vi "CVT2SaveAndReadTest.vi"() -> (3 "Unit Test Framework Results":T1)   [LabVIEW 2013, in "UnitTests.lvlib"]
uses:
  UnitTests.lvlib
  <vilib>/utf/common/utf_test_result_troll.ctl
  <vilib>/utf/common/utf_test_result.ctl
  <vilib>/utf/common/utf_test_result_failure.ctl
  <vilib>/utf/common/utf_test_comparison_operators.ctl
  <vilib>/utf/common/utf_vi_tag.ctl
  <vilib>/NI/Current Value Table/DataTypes/I32_Read Index.vi
  <vilib>/NI/Current Value Table/DataTypes/I32_Write Index.vi
  <vilib>/NI/Current Value Table/Memory Block.vi
  <vilib>/NI/Current Value Table/DataTypes/I32_Memory Block.vi
  <vilib>/utf/NI_UnitTestFramework.lvlib
  <vilib>/NI/Current Value Table/Current Value Table.lvlib
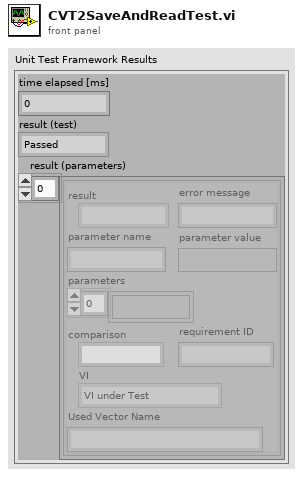
[diagram p1: front panel]
types:
  T1 = typedef "NI_UnitTestFramework.lvlib/utf_test_result_troll.ctl" = cluster{"time elapsed [ms]":u32, "result (test)":T2, "result (parameters)":T3[]}
  T2 = typedef "NI_UnitTestFramework.lvlib/utf_test_result.ctl" = enum16{"Passed", "Failed", "Error", "Skipped", "Not Processed"}
  T3 = typedef "NI_UnitTestFramework.lvlib/utf_test_result_failure.ctl" = cluster{"result":T2, "error message":string, "parameter name":string, "parameter value":variant, "parameters":variant[], "comparison":T4, "requirement ID":string, "VI":T5, "Used Vector Name":string}
  T4 = typedef "NI_UnitTestFramework.lvlib/utf_test_comparison_operators.ctl" = enum16{"=", "!=", ">", ">=", "<", "<=", "range", "symmetric tolerance", "asymmetric tolerance", "string contains", "string not contain", "array size", "string length", "array range", "by element", "array range (limit array)", "user-defined", "array contains", "array not contain", "vector length", "= (elm)", "!= (elm)", "= (case insensitive)", "!= (case insensitive)"}
  T5 = typedef "NI_UnitTestFramework.lvlib/utf_vi_tag.ctl" = enum16{"Setup VI", "VI under Test", "Teardown VI"}
  T6 = typedef "Current Value Table.lvlib/File Format.ctl" = cluster{"Tags":T7[], "Group Listings":T9[]}
  T7 = typedef "Current Value Table.lvlib/Single Tag.ctl" = cluster{"Data Type":T8, "Name":string, "Value":string, "Description":string}
  T8 = typedef "Current Value Table.lvlib/Data Types.ctl" = enum16{"Double", "Single", "I64", "I32", "I16", "I8", "U64", "U32", "U16", "U8", "String", "Boolean", "Array of U8", "Array of U16", "Array of U32", "Array of U64", "Array of I64", "Array of I32", "Array of I16", "Array of I8", "Array of Double", "Array of Single", "Array of Boolean", "Array of String"}
  T9 = typedef "Current Value Table.lvlib/Tag Grouping set.ctl" = cluster{"Group":string, "Tag Names":string[]}
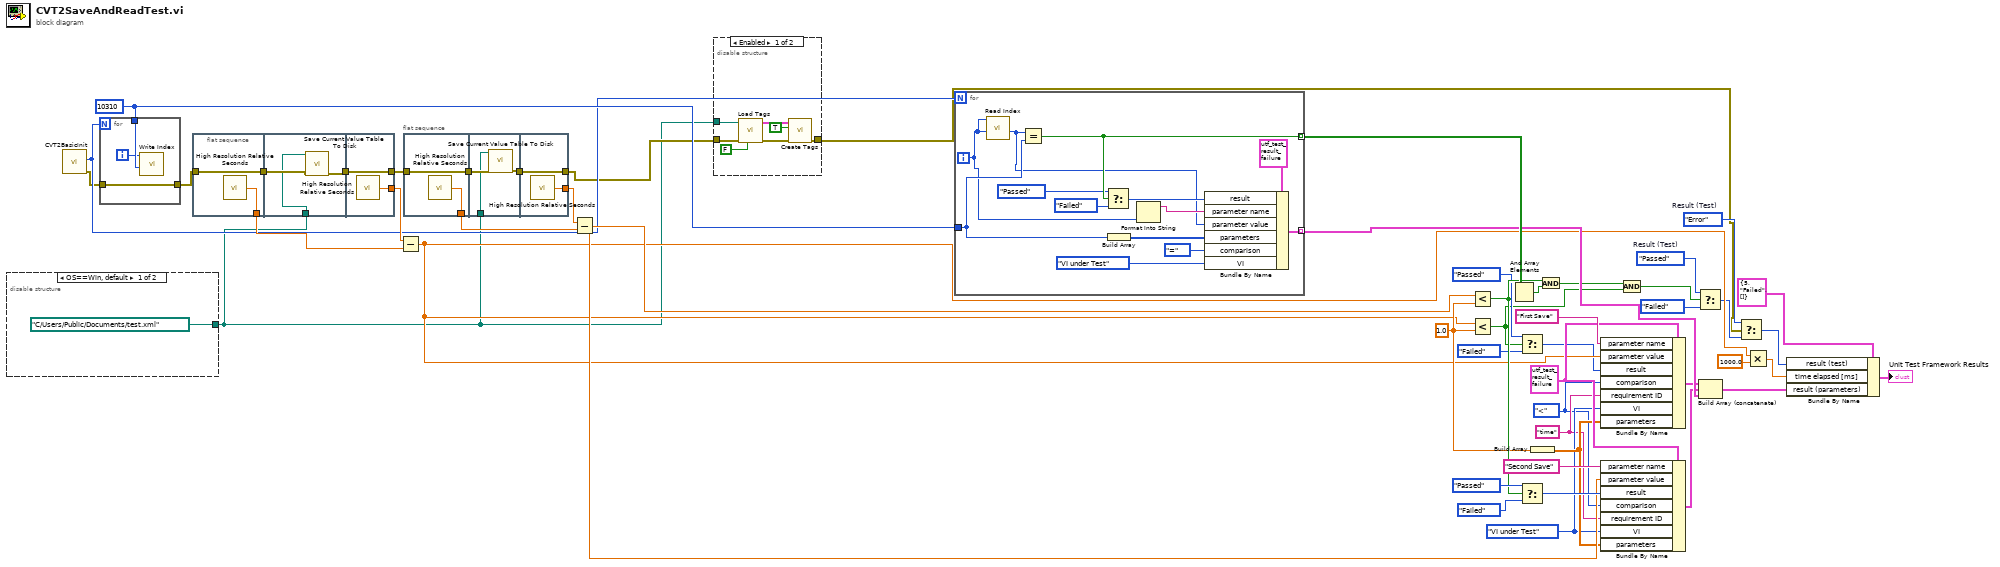
[diagram p0: block diagram]
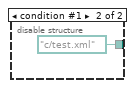
[diagram p3: hidden frame]
diagram:
  w29 = 10310 ("Value")
  w21 = T3 {"result"=enum."Passed", "error message"="", "parameter name"="", "parameter value"=variant, "parameters"=[], "comparison"=enum."=", "requirement ID"="", "VI"=enum."Setup VI", "Used Vector Name"=""} ("Unit Test Framework - result (parameters)")
  w26 = 1.0 ("y")
  w12 = "time" ("requirement ID")
  w11 = utf_test_comparison_operators."<" ("comparison")
  w13 = utf_vi_tag."VI under Test" ("VI")
  w48 = utf_test_result."Error"  # Result (Test)
  w8 = utf_test_result."Passed"  # Result (Test)
  n1 = disable-structure shown="OS==Win, default" {
    disable-tunnel: [path "C:/Users/Public/Documents/test.xml" ("XML File Path") path "c:/test.xml" ("XML File Path")] -> w4
    frame condition #0 (active) {
    }
    frame condition #1 {
    }
  }
  n2 = call "CVT2BasicInit.vi"() -> ("error out"=w1:errorcluster, "Tags per type out"=w10:i32)  [unwired: 9 in, 1 out]
  n3 = for {
    N: w10 -> [_]
    tunnel: w29 -> [w56]
    tunnel: [w54] -> w2
    tunnel: w1 -> [w54]
    i -> [w55]
    n4 = call-poly <vilib>:"Write Index.vi"("Value"=w56, "Index"=w55) -> ()  [unwired: 10 in]
  }
  n5 = flat-sequence {
    tunnel: w2 -> [w57]
    tunnel: [w57] -> w36
    tunnel: [w58] -> w34
    tunnel: [w61] -> w37
    tunnel: w36 -> [w60]
    tunnel: w4 -> [w59]
    tunnel: [w63] -> w30
    tunnel: w37 -> [w63]
    tunnel: [w62] -> w35
    frame #0 {
      n6 = call <vilib>:"High Resolution Relative Seconds.vi"() -> ("relative seconds"=w58:dbl)
    }
    frame #1 {
      n7 = call <vilib>:"Save Current Value Table To Disk.vi"("error in (no error)"=w60, "XML File Path"=w59) -> ("error out"=w61:errorcluster)  [unwired: 9 in]
    }
    frame #2 {
      n8 = call <vilib>:"High Resolution Relative Seconds.vi"() -> ("relative seconds"=w62:dbl)
    }
  }
  n9 = Subtract(x=w35, y=w34) -> (x-y=w19:dbl)
  n10 = flat-sequence {
    tunnel: w30 -> [w65]
    tunnel: [w65] -> w33
    tunnel: [w64] -> w32
    tunnel: w33 -> [w68]
    tunnel: w4 -> [w66]
    tunnel: [w67] -> w6
    tunnel: [w70] -> w5
    tunnel: [w69] -> w31
    tunnel: w6 -> [w70]
    frame #0 {
      n11 = call <vilib>:"High Resolution Relative Seconds.vi"() -> ("relative seconds"=w64:dbl)
    }
    frame #1 {
      n12 = call <vilib>:"Save Current Value Table To Disk.vi"("error in (no error)"=w68, "XML File Path"=w66) -> ("error out"=w67:errorcluster)  [unwired: 9 in]
    }
    frame #2 {
      n13 = call <vilib>:"High Resolution Relative Seconds.vi"() -> ("relative seconds"=w69:dbl)
    }
  }
  n14 = Subtract(x=w31, y=w32) -> (x-y=w20:dbl)
  n15 = disable-structure shown="Enabled" {
    disable-tunnel: w5 -> [w76 w78]
    disable-tunnel: w4 -> [w75 _]
    disable-tunnel: [w74 w78] -> w3
    frame Enabled {
      n16 = call <vilib>:"Load Tags.vi"("Create Tags? (T)"=FALSE, "error in (no error)"=w76, "XML File Path"=w75) -> ("error out"=w77:errorcluster, "CVT Tags"=w73:T6)  [unwired: 7 in]
      n17 = call <vilib>:"Create Tags.vi"("error in (no error)"=w77, "Clear Table? (F)"=TRUE, "CVT Tags to Create"=w73) -> ("error out"=w74:errorcluster)  [unwired: 8 in]
    }
    frame Disabled {
    }
  }
  n18 = for {
    N: w10 -> [_]
    tunnel: [w89] -> w45 mode=indexing
    tunnel: [w85] -> w39 mode=indexing
    tunnel: w29 -> [w81]
    i -> [w80]
    n19 = call-poly <vilib>:"Read Index.vi"("Default"=w80, "Index"=w80) -> ("Value"=w79:i32)  [unwired: 9 in]
    n20 = Equal?(x=w79, y=w81) -> (x = y?=w89:bool)
    n21 = Select(t=utf_test_result."Passed" ("result"), s=w89, f=utf_test_result."Failed" ("result")) -> (s? t:f=w86:T2)
    n22 = Build Array(w81) -> (w83:i32[])
    n23 = Format Into String(w80) -> (resulting string=w82:string)  [unwired: 3 in, 1 out]
    n24 = Bundle By Name(cluster=T3 {"result"=enum."Passed", "error message"="", "parameter name"="", "parameter value"=variant, "parameters"=[], "comparison"=enum."=", "requirement ID"="", "VI"=enum."Setup VI", "Used Vector Name"=""} ("Unit Test Framework - result (parameters)"), "result"=w86, "parameter name"=w82, "parameter value"=w79, "parameters"=w83, "comparison"=utf_test_comparison_operators."=", "VI"=utf_vi_tag."VI under Test") -> (w85:T3)
  }
  n25 = Less?(x=w20, y=w26) -> (x < y?=w38:bool)
  n26 = Less?(x=w19, y=w26) -> (x < y?=w15:bool)
  n27 = And Array Elements(Boolean array=w45) -> (logical AND=w44:bool)
  n28 = Select(t=utf_test_result."Passed" ("result"), s=w15, f=utf_test_result."Failed" ("result")) -> (s? t:f=w17:T2)
  n29 = Select(t=utf_test_result."Passed" ("result"), s=w38, f=utf_test_result."Failed" ("result")) -> (s? t:f=w42:T2)
  n30 = Build Array(w26) -> (w14:dbl[])
  n31 = And(x=w38, y=w44) -> (x .and. y?=w25:bool)
  n32 = Bundle By Name(cluster=w21, "parameter name"="First Save", "parameter value"=w19, "result"=w17, "comparison"=w11, "requirement ID"=w12, "VI"=w13, "parameters"=w14) -> (w23:T3)
  n33 = Bundle By Name(cluster=w21, "parameter name"="Second Save", "parameter value"=w20, "result"=w42, "comparison"=w11, "requirement ID"=w12, "VI"=w13, "parameters"=w14) -> (w28:T3)
  n34 = And(x=w25, y=w15) -> (x .and. y?=w24:bool)
  n35 = Select(t=w8, s=w24, f=utf_test_result."Failed") -> (s? t:f=w9:T2)
  n36 = Build Array (concatenate)(w23, w28, w39) -> (w27:T3[])
  n37 = Select(t=w48, s=w3, f=w9) -> (s? t:f=w7:T2)
  n38 = Multiply(x=w19, y=1000.0) -> (x*y=w46:dbl)
  n39 = Bundle By Name(cluster=T1 {"time elapsed [ms]"=5, "result (test)"=enum."Failed", "result (parameters)"=[]} ("Unit Test Framework - Result"), "result (test)"=w7, "time elapsed [ms]"=w46, "result (parameters)"=w27) -> (→"Unit Test Framework Results":T1)
